vi "ScanStop.vi"(11 "bar code scan":string) -> (1 "Boolean 3":bool, 2 "Boolean":bool, 3 "Boolean 2":bool)   [LabVIEW 2018]
panel:
  out "bar code scan 2":string
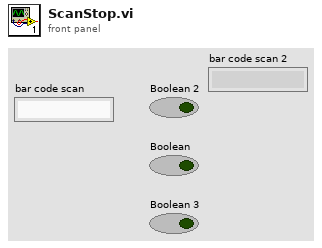
[diagram p1: front panel]
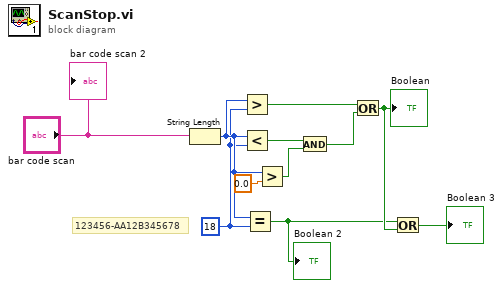
[diagram p0: block diagram]
diagram:
  w3 = 18
  # "123456-AA12B345678"
  n1 = String Length(string="bar code scan") -> (length=w4:i32)
  n2 = Greater?(x=w4, y=w3) -> (0:w7:bool)
  n3 = Less?(x=w4, y=w3) -> (x < y?=w6:bool)
  n4 = Equal?(x=w4, y=w3) -> (x = y?=w10:bool)
  "Boolean 2" <- w10
  n5 = Greater?(x=w4, y=0.0) -> (0:w5:bool)
  n6 = And(x=w6, y=w5) -> (x .and. y?=w8:bool)
  n7 = Or(x=w7, y=w8) -> (x .or. y?=w11:bool)
  "Boolean" <- w11
  n8 = Or(x=w10, y=w11) -> (x .or. y?=→"Boolean 3":bool)
  "bar code scan 2" <- "bar code scan"
